vi "Aktualizacja odległości.vi"(10 "Odległość od startu [m]":cluster{"X [m]":dbl, "Y [m]":dbl}, 11 "Lista współrzędnych":string[][](array[string])) -> (3 "Lista współrzędnych 2":string[][](array[string]))   [LabVIEW 2015, in "Biblioteka moduł map v3.lvlib" / "Obsługa listy współrzędnych.lvlib"]
doc: "Aktualizacja odległości do punktów docelowych na liście współrzędnych na podstawie znanej odległości robota od punktu startowego."
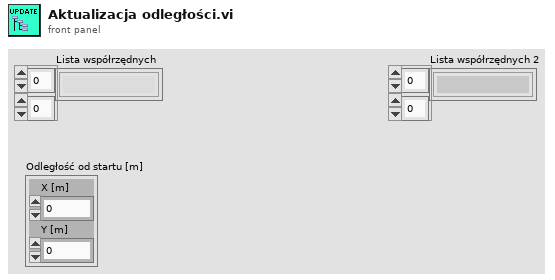
[diagram p1: front panel]
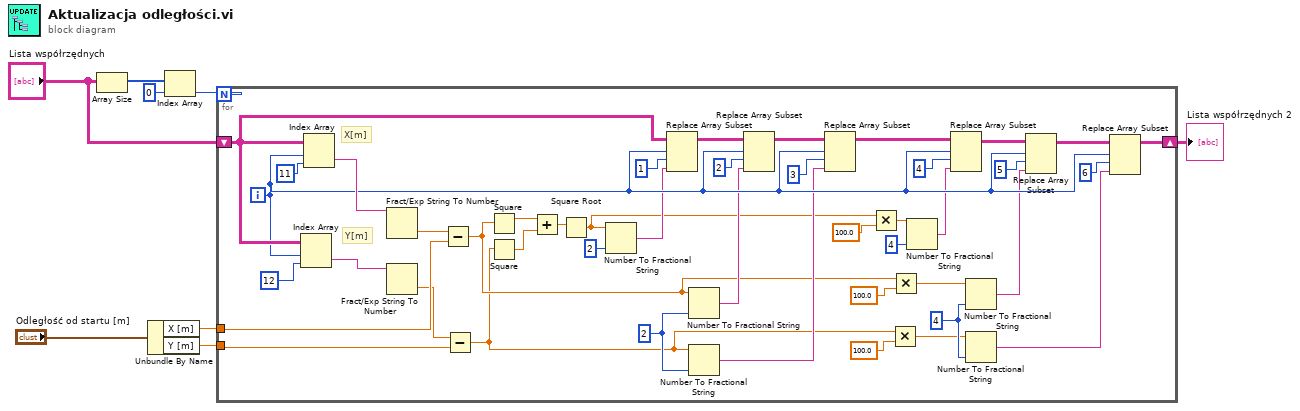
[diagram p0: block diagram]
diagram:
  n1 = Array Size(array="Lista współrzędnych") -> (size(s)=w8:i32[])
  n2 = Unbundle By Name("Odległość od startu [m]") -> ("X [m]"=w4:dbl, "Y [m]"=w3:dbl)
  n3 = Index Array(array=w8, index=0) -> (element=w6:i32)
  n4 = for {
    N: w6 -> [_]
    tunnel: w4 -> [w47]
    tunnel: w3 -> [w46]
    shift-right: [w45] -> w1
    shift-left: "Lista współrzędnych" -> [w39]
    i -> [w38]
    w17 = i16 4 ("precision (6)")
    w23 = i16 2 ("precision (6)")
    # "Y[m]"
    # "X[m]"
    n5 = Index Array(array=w39, index (row)=w38, index (col)=12 ("disabled index (col)")) -> (element=w50:string)
    n6 = Index Array(array=w39, index (row)=w38, index (col)=11 ("disabled index (col)")) -> (element=w49:string)
    n7 = Fract/Exp String To Number(string=w49) -> (number=w48:dbl)  [unwired: 3 in, 1 out]
    n8 = Fract/Exp String To Number(string=w50) -> (number=w30:dbl)  [unwired: 3 in, 1 out]
    n9 = Subtract(x=w48, y=w47) -> (x-y=w16:dbl)
    n10 = Subtract(x=w30, y=w46) -> (x-y=w15:dbl)
    n11 = Square(x=w16) -> (x^2=w28:dbl)
    n12 = Square(x=w15) -> (x^2=w27:dbl)
    n13 = Add(x=w28, y=w27) -> (x+y=w26:dbl)
    n14 = Square Root(x=w26) -> (sqrt(x)=w22:dbl)
    n15 = Number To Fractional String(number=w22, precision (6)=i16 2) -> (F-format string=w25:string)  [unwired: 2 in]
    n16 = Replace Array Subset(array=w39, new element=w25, index (row)=w38, index (col)=1 ("disabled index (col)")) -> (w40:string[][])
    n17 = Number To Fractional String(number=w16, precision (6)=w23) -> (F-format string=w31:string)  [unwired: 2 in]
    n18 = Number To Fractional String(number=w15, precision (6)=w23) -> (F-format string=w29:string)  [unwired: 2 in]
    n19 = Replace Array Subset(array=w40, new element=w31, index (row)=w38, index (col)=2 ("disabled index (col)")) -> (w41:string[][])
    n20 = Replace Array Subset(array=w41, new element=w29, index (row)=w38, index (col)=3 ("disabled index (col)")) -> (w42:string[][])
    n21 = Multiply(x=w22, y=100.0) -> (x*y=w21:dbl)
    n22 = Multiply(x=w15, y=100.0) -> (x*y=w13:dbl)
    n23 = Multiply(x=w16, y=100.0) -> (x*y=w14:dbl)
    n24 = Number To Fractional String(number=w21, precision (6)=i16 4) -> (F-format string=w19:string)  [unwired: 2 in]
    n25 = Replace Array Subset(array=w42, new element=w19, index (row)=w38, index (col)=4 ("disabled index (col)")) -> (w43:string[][])
    n26 = Number To Fractional String(number=w14, precision (6)=w17) -> (F-format string=w10:string)  [unwired: 2 in]
    n27 = Number To Fractional String(number=w13, precision (6)=w17) -> (F-format string=w9:string)  [unwired: 2 in]
    n28 = Replace Array Subset(array=w43, new element=w10, index (row)=w38, index (col)=5 ("disabled index (col)")) -> (w44:string[][])
    n29 = Replace Array Subset(array=w44, new element=w9, index (row)=w38, index (col)=6 ("disabled index (col)")) -> (w45:string[][])
  }
  "Lista współrzędnych 2" <- w1
